vi "HumanActionCache.vi"(7 "State":i32, 8 "Right X":dbl, 9 "Right Y":dbl, 10 "Left X":dbl, 11 "Left Y":dbl) -> (2 "RightMotorDemand":dbl, 3 "LeftMotorDemand":dbl)   [LabVIEW 2020]
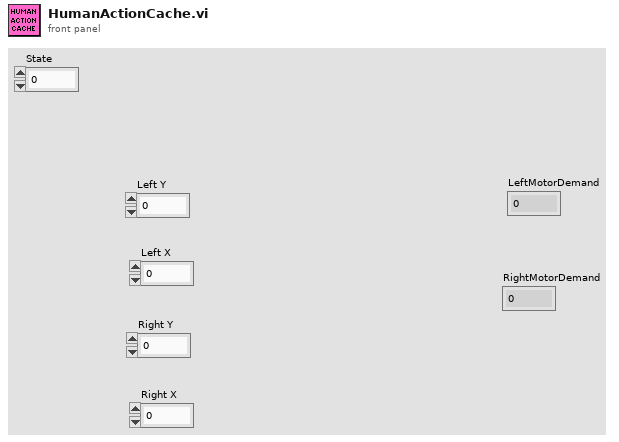
[diagram p1: front panel]
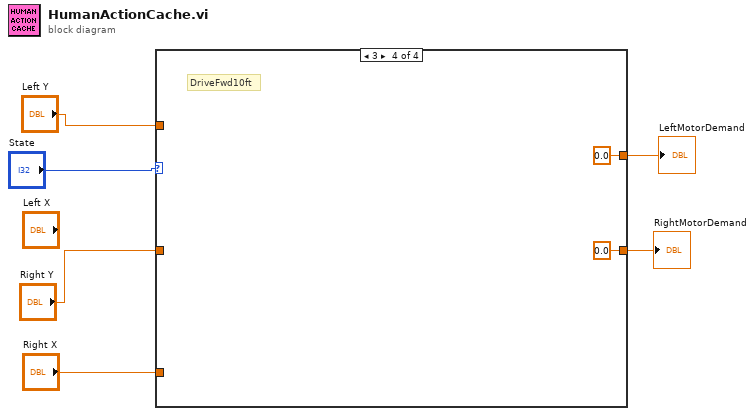
[diagram p0: block diagram]
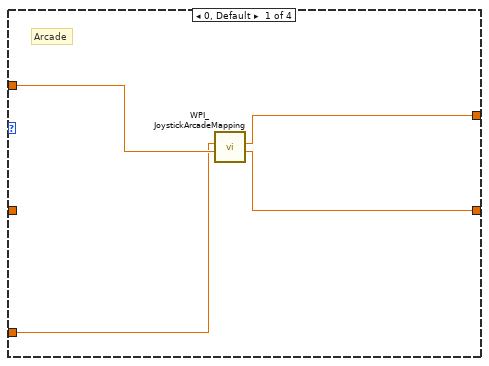
[diagram p2: hidden frame]
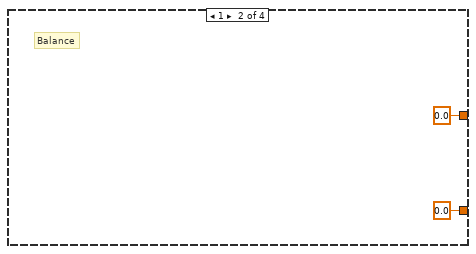
[diagram p3: hidden frame]
diagram:
  n1 = case shown="3" "State" {
    tunnel: "Left Y" -> [w10 _ w14 _]
    tunnel: "Right X" -> [w9 _ _ _]
    tunnel: [w8 0.0 ("Left Y") w14 0.0 ("Left Y")] -> w4
    tunnel: [w7 0.0 ("Right Y") w13 0.0 ("Right Y")] -> w3
    tunnel: "Right Y" -> [_ _ w13 _]
    frame 0, Default {
      # "Arcade"
      n2 = call <vilib>:"WPI_JoystickArcadeMapping.vi"("Y axis value"=w10, "X axis value"=w9) -> ("Right Motor Value"=w7:dbl, "Left Motor Value"=w8:dbl)  [unwired: 8 in]
    }
    frame 1 {
      # "Balance"
    }
    frame 2 {
      # "Tank"
    }
    frame 3 {
      # "DriveFwd10ft"
    }
  }
  "LeftMotorDemand" <- w4
  "RightMotorDemand" <- w3
